vi "GUI controls.vi"(0 "Edit":refnum<vi>, 5 "Delete":refnum<vi>, 7 "Design":refnum<vi>, 9 "Project List":refnum<vi>, 11 "error in (no error)":errorcluster, 12 "GUI controls commands":T1) -> (15 "error out":errorcluster)   [LabVIEW 2015]
uses:
  GUI controls commands.ctl
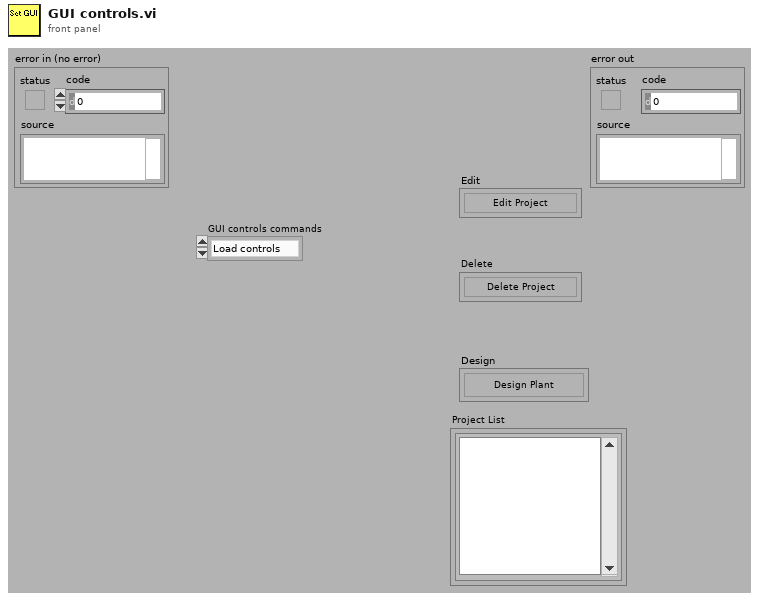
[diagram p1: front panel]
types:
  T1 = typedef "GUI controls commands.ctl" = enum16{"Load controls", "Set controls"}
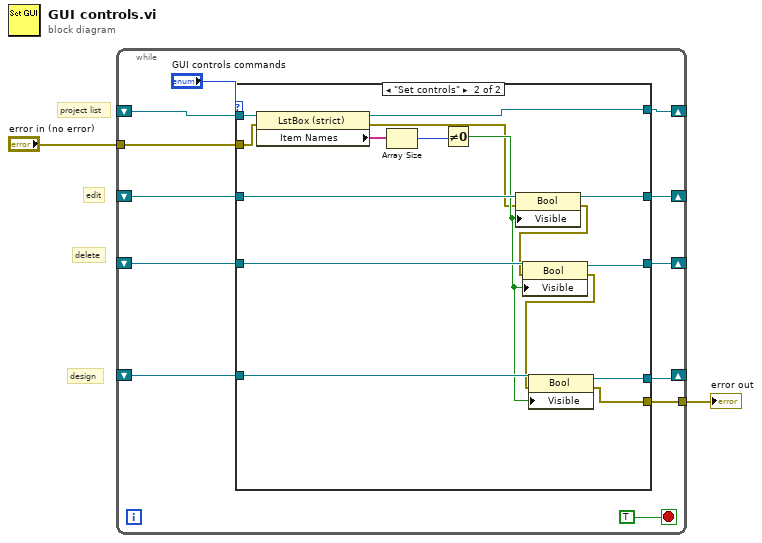
[diagram p0: block diagram]
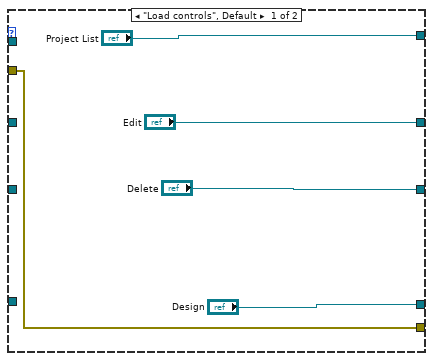
[diagram p2: hidden frame]
diagram:
  # "project list"
  # "design"
  # "delete"
  # "edit"
  n1 = while {
    shift-right: [w13] -> _
    shift-left: _ -> [w9]
    shift-right: [w12] -> _
    shift-left: _ -> [w8]
    shift-right: [w11] -> _
    shift-left: _ -> [w7]
    shift-right: [w10] -> _
    shift-left: _ -> [w6]
    tunnel: [w4] -> w2
    tunnel: "error in (no error)" -> [w3]
    stop <- TRUE stop-if-true
    n2 = case shown="\"Set controls\"" "GUI controls commands" {
      tunnel: ["Edit" w27] -> w13
      tunnel: ["Delete" w28] -> w12
      tunnel: ["Design" w30] -> w11
      tunnel: ["Project List" w34] -> w10
      tunnel: w9 -> [_ w32]
      tunnel: w8 -> [_ w29]
      tunnel: w7 -> [_ w31]
      tunnel: w6 -> [_ w35]
      tunnel: [w15 w22] -> w4
      tunnel: w3 -> [w15 w21]
      frame "Load controls", Default {
      }
      frame "Set controls" {
        n3 = property class="LstBox (strict)"(reference=w35, error in=w21) -> (reference out=w34:refnum<vi>, error out=w25:errorcluster, "Item Names"=w33:string[])
        n4 = Array Size(array=w33) -> (size(s)=w20:i32)
        n5 = Not Equal To 0?(x=w20) -> (x != 0?=w26:bool)
        n6 = property class="Bool"(reference=w32, error in=w25, "Visible"=w26) -> (reference out=w27:refnum<vi>, error out=w24:errorcluster)
        n7 = property class="Bool"(reference=w29, error in=w24, "Visible"=w26) -> (reference out=w28:refnum<vi>, error out=w23:errorcluster)
        n8 = property class="Bool"(reference=w31, error in=w23, "Visible"=w26) -> (reference out=w30:refnum<vi>, error out=w22:errorcluster)
      }
    }
  }
  "error out" <- w2
